vi "Sub_Check_MAC_address.vi"() -> ()   [LabVIEW 2015]
panel:
  in  "문자열":string="DA:29:F7:1B:EE:B5"
  out "Check Count":i32
  in  "Device List":i32(listbox)=2
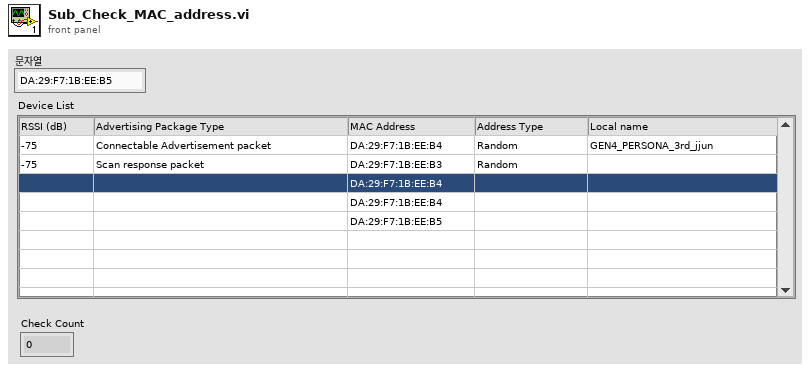
[diagram p1: front panel]
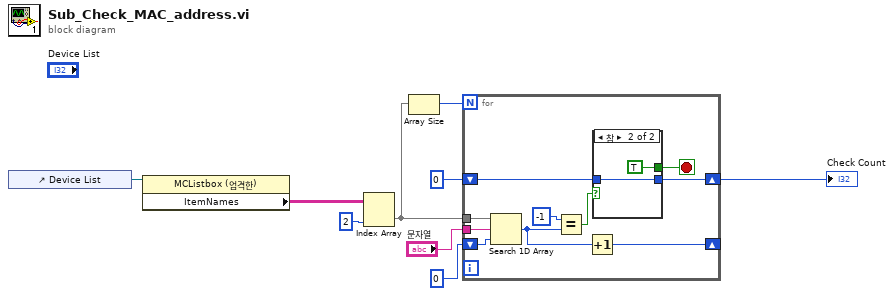
[diagram p0: block diagram]
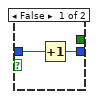
[diagram p2: hidden frame]
diagram:
  n1 = control-ref of="Device List"() -> (w7:refnum<vi>)
  n2 = property class="MCListbox (엄격한)"(reference=w7) -> ("ItemNames"=w9:string[][])  [unwired: 1 in, 2 out]
  n3 = Index Array(array=w9, index (col)=2 ("비활성화된 인덱스 (열)")) -> (element=w5:string[])  [unwired: 1 in]
  n4 = Array Size(array=w5) -> (size(s)=w4:i32)
  n5 = for {
    N: w4 -> [_]
    tunnel: w5 -> [w19]
    tunnel: "문자열" -> [w18]
    shift-right: [w14] -> _
    shift-left: 0 ("index of element") -> [w15]
    shift-right: [w16] -> w1
    shift-left: 0 ("index of element") -> [w17]
    stop <- w10 stop-if-true
    n6 = Search 1D Array(1D array=w19, element=w18, start index (0)=w15) -> (index of element=w13:i32)
    n7 = Equal?(x=-1, y=w13) -> (x = y?=w12:bool)
    n8 = Increment(x=w13) -> (x+1=w14:i32)
    n9 = case shown="참" w12 {
      tunnel: w17 -> [w21 w23]
      tunnel: [w20 w23] -> w16
      tunnel: [_ TRUE] -> w10
      frame False {
        n10 = Increment(x=w21) -> (x+1=w20:i32)
      }
      frame True {
      }
    }
  }
  "Check Count" <- w1
